vi "Close.vi"(8 "error in (no error)":errorcluster, 11 "LCD in":refnum<class "Character LCD.lvclass">) -> (0 "error out":errorcluster)   [LabVIEW 2017, in "HD44780 Host.lvlib"]
doc: "ORIGINAL CODE: \nBy: National Instruments\n NI LabVIEW RIO Evaluation Kit\n Code example \"5- Startup Application\"\n www.ni.com/embeddedsystems\n\nUPDATED CODE: Adds NI SystemLink and NI AWS LabVIEW Tookit functionality for demonstration. \nBy: James Tillett\n Endeavor Engineering Inc.\n www.endeavoreng.com"
uses:
  HD44780 Host.lvlib
  Internal/LCD Class/Character LCD.lvclass
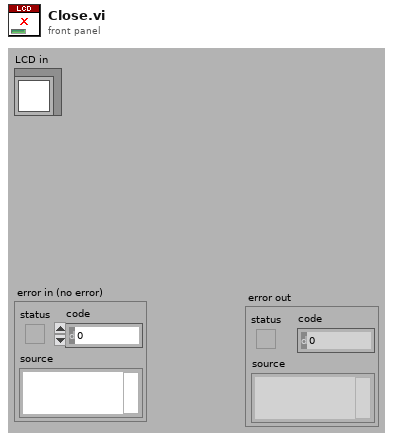
[diagram p1: front panel]
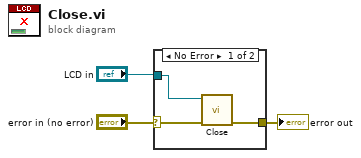
[diagram p0: block diagram]
diagram:
  n1 = case shown="No Error" "error in (no error)" {
    selector: "error in (no error)" -> [w6 w7]
    tunnel: [w5 w7] -> w1
    tunnel: "LCD in" -> [w4 _]
    frame No Error {
      n2 = call-dynamic "Close.vi"("error in (no error)"=w6, "Character LCD in"=w4) -> ("error out"=w5:errorcluster)  [unwired: 9 in]
    }
    frame Error {
    }
  }
  "error out" <- w1
